vi "VSSDetectionFIRASimFrame.vi"(8 "error in (no error)":errorcluster, 9 "FIRASim?":bool, 11 "Frame":u8[](array[numeric])) -> (0 "error out":errorcluster, 3 "Detection Frame out":T1 {"robots_blue"."height" format="%+4.3f"; "robots_blue"."pixel_y" format="%+4.3f"; "robots_blue"."pixel_x" format="%+4.3f"; "robots_blue"."orientation" format="%+4.3f"; "robots_blue"."y" format="%+4.3f"; "robots_blue"."confidence" format="%4.3f"; "robots_blue"."x" format="%+4.3f"; "robots_yellow"."height" format="%+4.3f"; "robots_yellow"."pixel_y" format="%+4.3f"; "robots_yellow"."pixel_x" format="%+4.3f"; "robots_yellow"."orientation" format="%+4.3f"; "robots_yellow"."y" format="%+4.3f"; "robots_yellow"."confidence" format="%4.3f"; "robots_yellow"."x" format="%+4.3f"})   [LabVIEW 2020]
uses:
  Controls/SSL Detection Frame.ctl
  Controls/SSL Detection Robot.ctl
  <vilib>/Analysis/Matrix/Datatypes/RealMatrix.ctl
  Controls/SSL Detection Ball.ctl
  <vilib>/Analysis/Matrix/NI_Matrix.lvlib
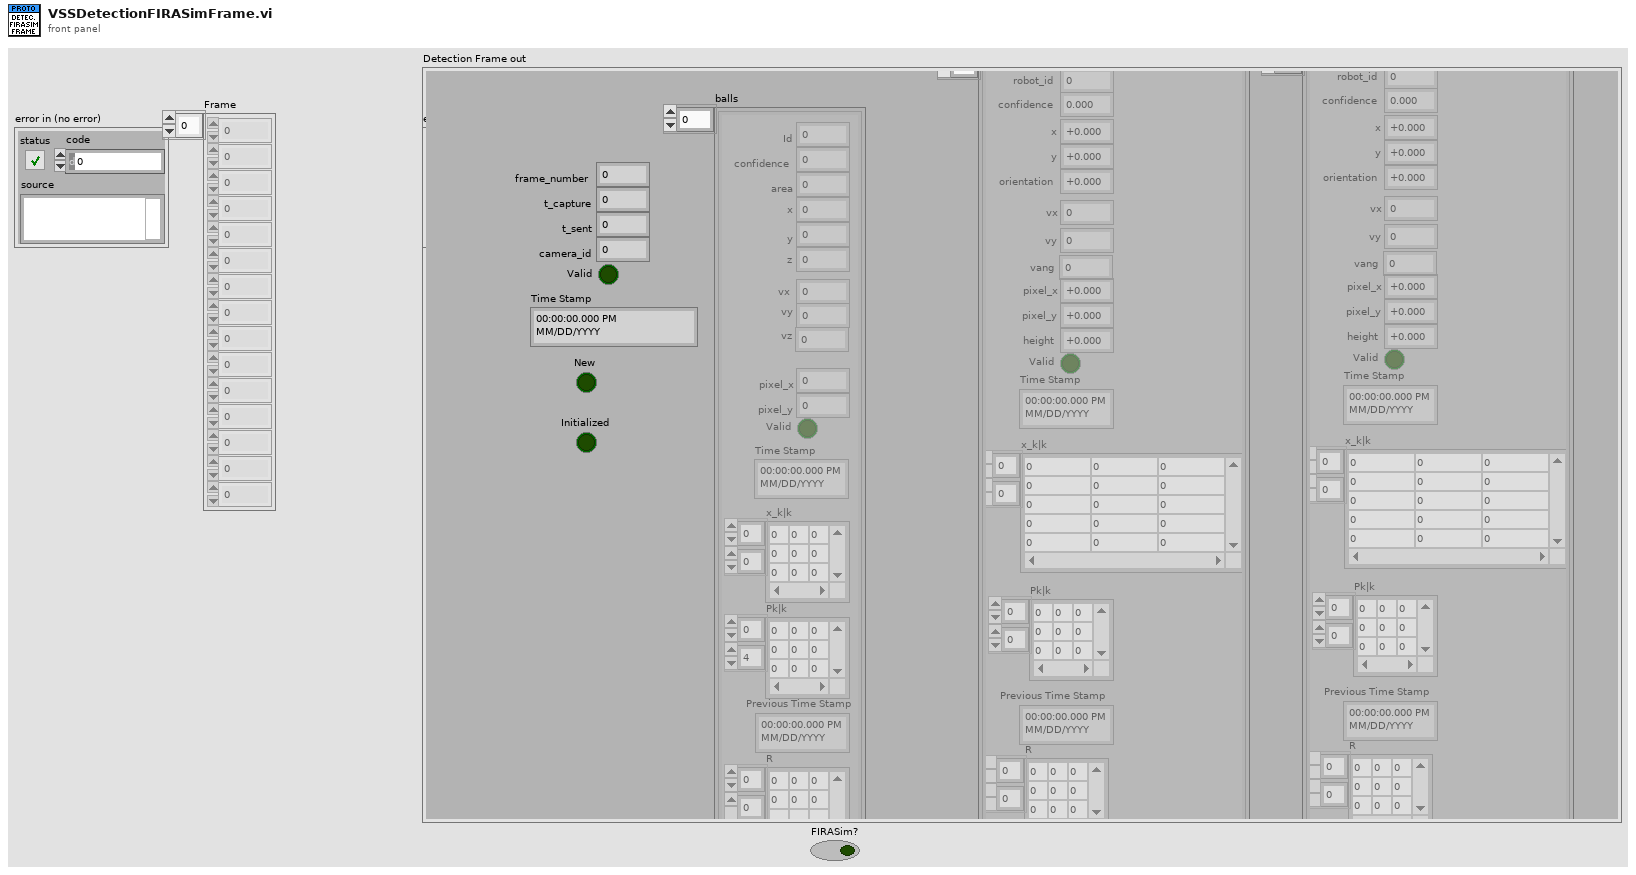
[diagram p1: front panel]
types:
  T1 = typedef "SSL Detection Frame.ctl" = cluster{"frame_number":u32, "t_capture":dbl, "t_sent":dbl, "camera_id":u32, "robots_yellow":T2[], "robots_blue":T2[], "balls":T4[], "Valid":bool, "Time Stamp":timestamp, "New":bool, "Initialized":bool}
  T2 = typedef "SSL Detection Robot.ctl" = cluster{"x":sgl, "robot_id":u32, "confidence":sgl, "y":sgl, "orientation":sgl, "pixel_x":sgl, "pixel_y":sgl, "height":sgl, "Valid":bool, "Time Stamp":timestamp, "x_k|k":T3, "Pk|k":T3, "Previous Time Stamp":timestamp, "R":T3, "vx":dbl, "vy":dbl, "vang":dbl}
  T3 = typedef "NI_Matrix.lvlib/RealMatrix.ctl" = dbl[][]
  T4 = typedef "SSL Detection Ball.ctl" = cluster{"x":sgl, "area":u32, "confidence":sgl, "y":sgl, "z":sgl, "pixel_x":sgl, "pixel_y":sgl, "Valid":bool, "Time Stamp":timestamp, "x_k|k":T3, "Pk|k":T3, "Id":u32, "Previous Time Stamp":timestamp, "R":T3, " vx":sgl, "vy":dbl, "vz":dbl}
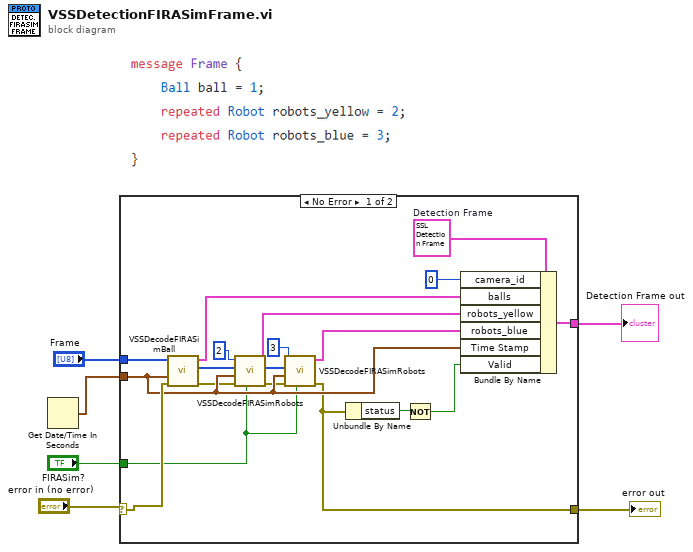
[diagram p0: block diagram]
diagram:
  n1 = Get Date/Time In Seconds() -> (seconds since 1Jan1904=w3:timestamp)
  n2 = case shown="No Error" "error in (no error)" {
    selector: "error in (no error)" -> [w12 w26]
    tunnel: "Frame" -> [w25 _]
    tunnel: [w7 w26] -> w4
    tunnel: w3 -> [w11 _]
    tunnel: [w19 _] -> w2
    tunnel: "FIRASim?" -> [w10 _]
    frame No Error {
      w23 = T1 {"frame_number"=0, "t_capture"=0.0, "t_sent"=0.0, "camera_id"=0, "robots_yellow"=[], "robots_blue"=[], "balls"=[], "Valid"=FALSE, "Time Stamp"=timestamp(0 s since 1904-01-01), "New"=FALSE, "Initialized"=FALSE}  # Detection Frame
      n3 = call "VSSDecodeFIRASimBall.vi"("error in (no error)"=w12, "TimeStamp"=w11, "Frame"=w25) -> ("error out"=w9:errorcluster, "Robots"=w18:u8[], "Balls out"=w22:T4[])  [unwired: 6 in]
      n4 = call "VSSDecodeFIRASimRobots.vi"("FIRASim?"=w10, "error in"=w9, "Time Stamp"=w11, "Robots"=w18, "Key"=2) -> ("error out"=w8:errorcluster, "array w/ subset deleted out"=w17:u8[], "Robots"=w21:T2[])  [unwired: 4 in]
      n5 = call "VSSDecodeFIRASimRobots.vi"("FIRASim?"=w10, "error in"=w8, "Time Stamp"=w11, "Robots"=w17, "Key"=3) -> ("error out"=w7:errorcluster, "Robots"=w15:T2[])  [unwired: 4 in, 1 out]
      n6 = Unbundle By Name(w7) -> ("status"=w14:bool)
      n7 = Not(x=w14) -> (.not. x?=w13:bool)
      n8 = Bundle By Name(cluster=w23, "camera_id"=u32 0, "balls"=w22, "robots_yellow"=w21, "robots_blue"=w15, "Time Stamp"=w11, "Valid"=w13) -> (w19:T1)
    }
    frame Error {
    }
  }
  "error out" <- w4
  "Detection Frame out" <- w2
